vi "packBool2ChImToU32.vi"(1 "ch1":bool[](array[boolean]), 2 "ch0":bool[](array[boolean])) -> (0 "buffer":u32[](array[numeric]))   [LabVIEW 2010]
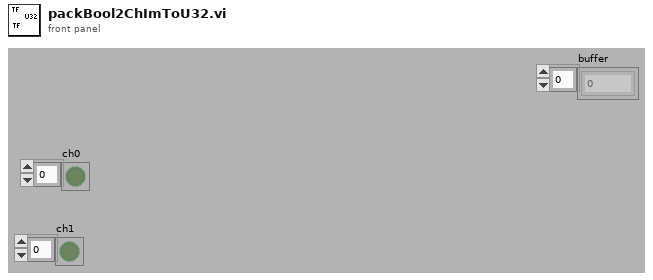
[diagram p1: front panel]
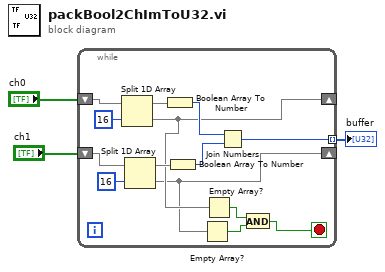
[diagram p0: block diagram]
diagram:
  n1 = while {
    shift-right: [w8] -> _
    shift-left: "ch0" -> [w17]
    shift-right: [w7] -> _
    shift-left: "ch1" -> [w12]
    tunnel: [w9] -> w1 mode=indexing
    stop <- w4 stop-if-true
    n2 = Split 1D Array(array=w17, index=16) -> (first subarray=w15:bool[], second subarray=w8:bool[])
    n3 = Split 1D Array(array=w12, index=16) -> (first subarray=w13:bool[], second subarray=w7:bool[])
    n4 = Boolean Array To Number(Boolean array=w15) -> (number=w11:u16)
    n5 = Boolean Array To Number(Boolean array=w13) -> (number=w10:u16)
    n6 = Empty Array?(array=w7) -> (empty?=w5:bool)
    n7 = Empty Array?(array=w8) -> (empty?=w6:bool)
    n8 = Join Numbers(hi=w11, lo=w10) -> ((hi.lo)=w9:u32)
    n9 = And(x=w6, y=w5) -> (x .and. y?=w4:bool)
  }
  "buffer" <- w1
